vi "FTW-Context-NewLoggerConnection.vi"(5 "Logger Address":string, 11 "error in":errorcluster) -> (4 "Event Logger Connection":refnum<class "FTW-Logger.lvclass">, 15 "error out":errorcluster)   [LabVIEW 2013, in "FTW-Actor-Context.lvclass"]
uses:
  FTW-Actor-Context.lvclass
  logger/FTW-Logger.lvclass
  FTW-Context-Instance.vi
panel:
  # "Inputs"
  # "Outputs"
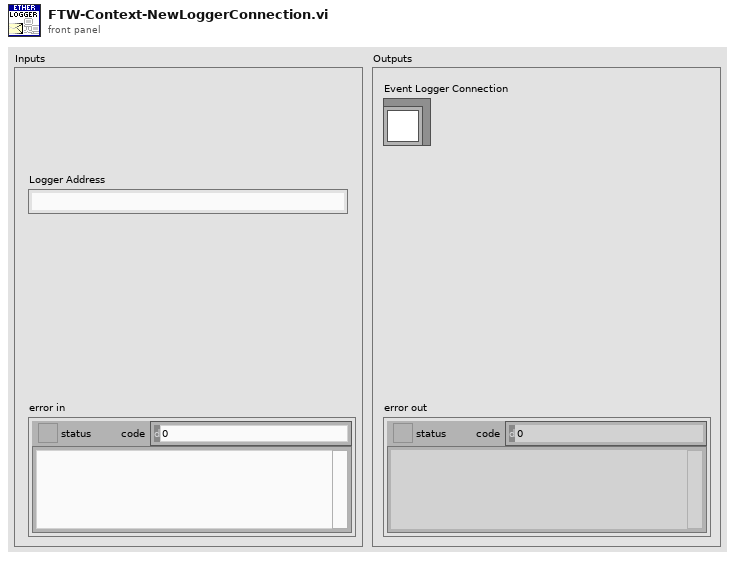
[diagram p1: front panel]
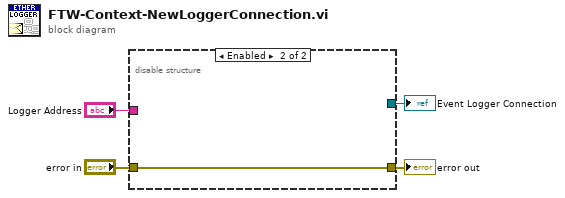
[diagram p0: block diagram]
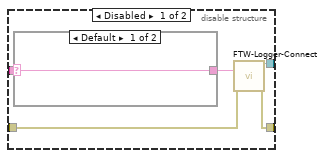
[diagram p2: hidden frame]
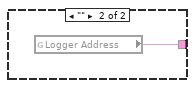
[diagram p3: hidden frame]
diagram:
  n1 = disable-structure shown="Enabled" {
    disable-tunnel: "error in" -> [w9 w12]
    disable-tunnel: [w8 w12] -> w3
    disable-tunnel: [w7 _] -> w2
    disable-tunnel: "Logger Address" -> [w5 _]
    frame Disabled {
      n2 = case shown="Default" w5 {
        selector: w5 -> [w10 _]
        tunnel: [w10 w11] -> w6
        frame Default {
        }
        frame "" {
          n3 = global read "FTW-Context-Instance.vi" "Logger Address"() -> (w11:string)
        }
      }
      n4 = call "FTW-Logger-Connect.vi"("Logger Address"=w6, "error in"=w9) -> ("FTW Logger Connector"=w7:refnum<class "FTW-Logger.lvclass">, "error out"=w8:errorcluster)  [unwired: 12 in]
    }
    frame Enabled {
    }
  }
  "error out" <- w3
  "Event Logger Connection" <- w2
